vi "SingleAcquisitionDisplayImageData.vi"() -> ()   [LabVIEW 2018]
uses:
  C:/Users/dyoshida/Documents/__labview/________phase_3_final/LabVIEWSamples/Release/Dependencies/PVCamNET.dll
  Dependencies/PVCamNET.dll
panel:
  out "Min":dbl
  out "Max":dbl
  out "RawImageData":i32[](array[numeric])
  out "Waveform Graph":i32[](graph)
  out "Boolean 2":bool
  out "Boolean":bool
  in  "?":bool
  in  "?":bool
  in  "Exposure time":dbl=30.0
  in  "?":bool
  # "SingleAcquisitionDisplayImageData.vi\n\nDescription:\nThis sample code lets the user access the image data from the buffer.\n\nSteps to run:\n1. Click \"Run\"\n2. Enter exposure time\n3. Click \"START\"\n4. Click \"DISPLAY\"\n5. Click \"CLOSE\""
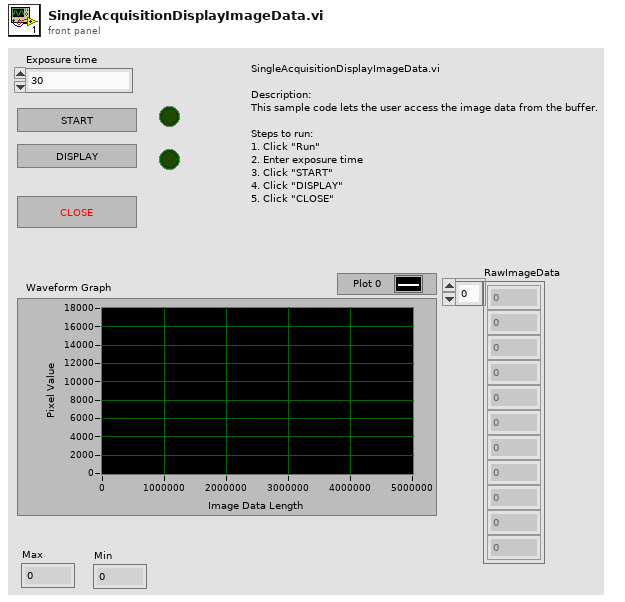
[diagram p1: front panel]
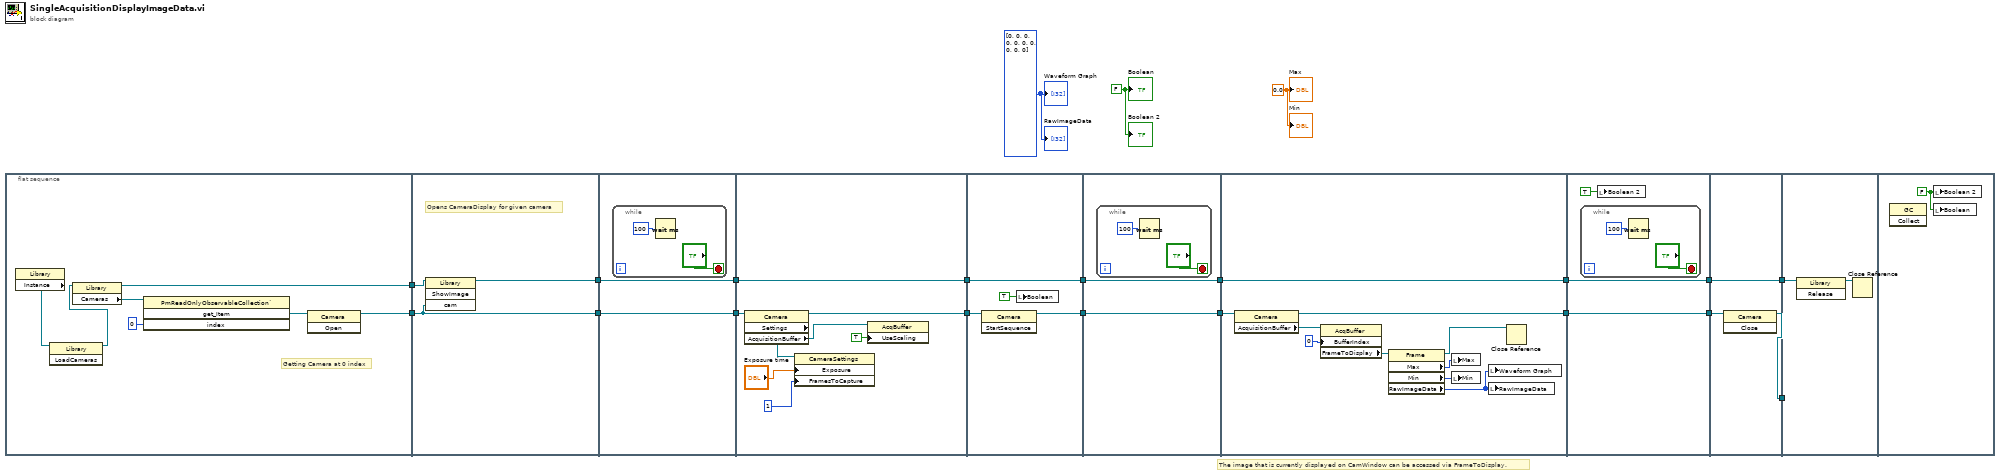
[diagram p0: block diagram]
diagram:
  w1 = 0.0 ("Max")
  w2 = i32[] [0, 0, 0, 0, 0, 0, 0, 0, 0, 0] ("RawImageData")
  w5 = FALSE ("Boolean")
  # "The image that is currently displayed on CamWindow can be accessed via FrameToDisplay."
  n1 = flat-sequence {
    tunnel: [w24] -> w21
    tunnel: [w25] -> w20
    tunnel: w21 -> [w31]
    tunnel: w20 -> [w30]
    tunnel: [w30] -> w19
    tunnel: [w29] -> w18
    tunnel: w19 -> [w33]
    tunnel: [w33] -> w16
    tunnel: w18 -> [w32]
    tunnel: [w32] -> w17
    tunnel: [w43] -> w15
    tunnel: [w42] -> w14
    tunnel: w17 -> [w42]
    tunnel: w16 -> [w41]
    tunnel: w15 -> [w46]
    tunnel: [w45] -> w9
    tunnel: [w47] -> w7
    tunnel: w14 -> [w47]
    tunnel: w9 -> [w49]
    tunnel: [w49] -> w8
    tunnel: w7 -> [w48]
    tunnel: [w48] -> w6
    tunnel: w8 -> [w60]
    tunnel: [w57] -> w4
    tunnel: w6 -> [w61]
    tunnel: [w61] -> w3
    tunnel: w4 -> [w64]
    tunnel: [w64] -> w11
    tunnel: w3 -> [w63]
    tunnel: [w63] -> w10
    tunnel: w11 -> [w69]
    tunnel: w10 -> [w67]
    tunnel: [w68] -> w13
    tunnel: [w67] -> w12
    tunnel: w13 -> [_]
    tunnel: w12 -> [w71]
    frame #0 {
      # "Getting Camera at 0 index"
      n2 = property class="Library"() -> ("Instance"=w23:refnum<k24>)  [unwired: 2 in, 2 out]
      n3 = invoke class="Library" method="LoadCameras"(reference=w23) -> (reference out=w22:refnum<k24>)  [unwired: 2 in, 2 out]
      n4 = property class="Library"(reference=w22) -> (reference out=w24:refnum<k24>, "Cameras"=w28:refnum<k24>)  [unwired: 1 in, 1 out]
      n5 = invoke class="PmReadOnlyObservableCollection`" method="get_Item"(reference=w28, "index"=0) -> ("get_Item"=w26:refnum<k24>)  [unwired: 2 in, 3 out]
      n6 = invoke class="Camera" method="Open"(reference=w26) -> (reference out=w25:refnum<k24>)  [unwired: 2 in, 2 out]
    }
    frame #1 {
      # "Opens CameraDisplay for given camera"
      n7 = invoke class="Library" method="ShowImage"(reference=w31, "cam"=w30) -> (reference out=w29:refnum<k24>)  [unwired: 2 in, 3 out]
    }
    frame #2 {
      n8 = while {
        stop <- "?" stop-if-true
        n9 = Wait (ms)(milliseconds to wait=u32 100) -> ()  [unwired: 1 out]
      }
    }
    frame #3 {
      n10 = property class="Camera"(reference=w41) -> (reference out=w43:refnum<k24>, "Settings"=w39:refnum<k24>, "AcquisitionBuffer"=w37:refnum<k24>)  [unwired: 1 in, 1 out]
      n11 = property class="CameraSettings"(reference=w39, "Exposure"="Exposure time", "FramesToCapture"=u16 1) -> ()  [unwired: 1 in, 2 out]
      n12 = property class="AcqBuffer"(reference=w37, "UseScaling"=TRUE) -> ()  [unwired: 1 in, 2 out]
    }
    frame #4 {
      n13 = invoke class="Camera" method="StartSequence"(reference=w46) -> (reference out=w45:refnum<k24>)  [unwired: 2 in, 2 out]
      n14 = local write "Boolean"(TRUE ("Boolean")) -> ()
    }
    frame #5 {
      n15 = while {
        stop <- "?" stop-if-true
        n16 = Wait (ms)(milliseconds to wait=u32 100) -> ()  [unwired: 1 out]
      }
    }
    frame #6 {
      n17 = property class="Camera"(reference=w60) -> (reference out=w57:refnum<k24>, "AcquisitionBuffer"=w59:refnum<k24>)  [unwired: 1 in, 1 out]
      n18 = property class="AcqBuffer"(reference=w59, "BufferIndex"=0) -> ("FrameToDisplay"=w54:refnum<k24>)  [unwired: 1 in, 2 out]
      n19 = property class="Frame"(reference=w54) -> (reference out=w52:refnum<k24>, "Max"=w56:u32, "Min"=w55:u32, "RawImageData"=w53:i16[])  [unwired: 1 in, 1 out]
      n20 = local write "Max"(w56) -> ()
      n21 = local write "Min"(w55) -> ()
      n22 = local write "Waveform Graph"(w53) -> ()
      n23 = local write "RawImageData"(w53) -> ()
      n24 = Close Reference(reference=w52) -> ()  [unwired: 1 in, 1 out]
    }
    frame #7 {
      n25 = while {
        stop <- "?" stop-if-true
        n26 = Wait (ms)(milliseconds to wait=u32 100) -> ()  [unwired: 1 out]
      }
      n27 = local write "Boolean 2"(TRUE ("Boolean 2")) -> ()
    }
    frame #8 {
      n28 = invoke class="Camera" method="Close"(reference=w69) -> (reference out=w68:refnum<k24>)  [unwired: 2 in, 2 out]
    }
    frame #9 {
      n29 = invoke class="Library" method="Release"(reference=w71) -> (reference out=w70:refnum<k24>)  [unwired: 2 in, 2 out]
      n30 = Close Reference(reference=w70) -> ()  [unwired: 1 in, 1 out]
    }
    frame #10 {
      w72 = FALSE ("Boolean 2")
      n31 = invoke class="GC" method="Collect"() -> ()  [unwired: 3 in, 3 out]
      n32 = local write "Boolean 2"(w72) -> ()
      n33 = local write "Boolean"(w72) -> ()
    }
  }
  "Boolean" <- w5
  "Boolean 2" <- w5
  "RawImageData" <- w2
  "Waveform Graph" <- w2
  "Max" <- w1
  "Min" <- w1
